vi "EF_GetFeaturesDecimate.vi"(8 "error in (no error)":errorcluster, 10 "Decimating Factor":i32=1, 11 "Array Of Waveforms in":waveform(dbl)[](array[waveform])) -> (0 "error out":errorcluster, 3 "Features Array out":dbl[][](array[numeric]))   [LabVIEW 2016, in "Feature Extraction.lvlib"]
uses:
  <vilib>/Analysis/2dsp.llb/Decimate (single shot, DBL).vi
  Feature Extraction.lvlib
  <vilib>/Analysis/NI_AALPro.lvlib
panel:
  out "Waveform Graph":dbl[][](graph)
  # "This VI is a part of BCI Design library, http://www.ru-bci.org \nCopyright © 2020, Sotnikov Peter, All rights reserved. License: GNU GPLv3"
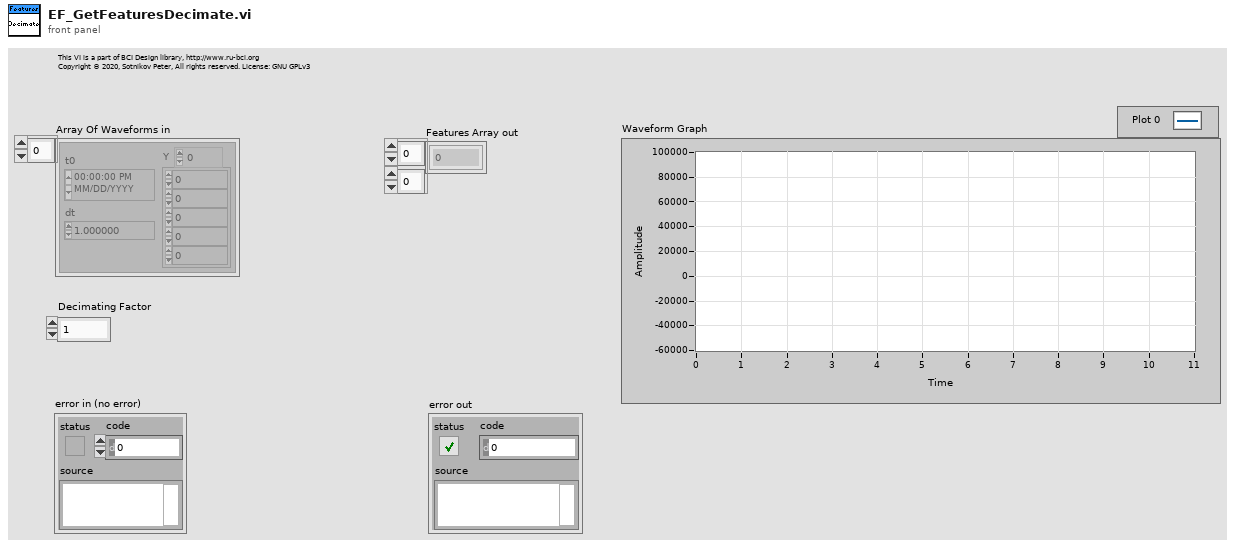
[diagram p1: front panel]
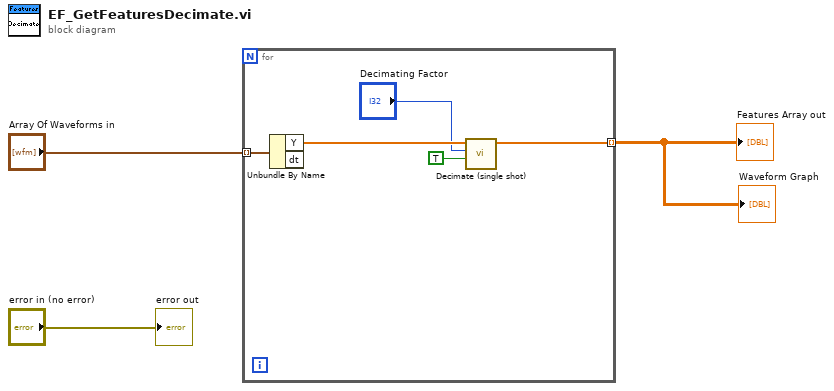
[diagram p0: block diagram]
diagram:
  n1 = for {
    tunnel: [w5] -> w3 mode=indexing
    tunnel: "Array Of Waveforms in" -> [w7] mode=indexing
    n2 = Unbundle By Name(w7) -> ("Y"=w6:dbl[])  [unwired: 1 out]
    n3 = call-poly <vilib>:"Decimate (single shot).vi"("averaging"=TRUE, "decimating factor"="Decimating Factor", "X"=w6) -> ("Decimated Array"=w5:dbl[])  [unwired: 7 in, 1 out]
  }
  "Features Array out" <- w3
  "Waveform Graph" <- w3
  "error out" <- "error in (no error)"
